vi "pixelfly_init.vi"(0 "trigger":bool=TRUE, 1 "V bin":i32(ring) items=["1", "2"], 2 "exp level":i32=1 min=0 max=255 step=1, 5 "Exposure mode":u16(ring)=1 items=["Asynch shutter", "Double shot", "Video mode", "Auto exposure"], 7 "exp time":i32=150 min=1 max=10000, 9 "gain":i32(ring) items=["Low (X1)", "High (X2)"], 11 "error in (no error)":errorcluster, 12 "H bin":i32(ring) items=["1", "2"]) -> (3 "X Bin":i32, 4 "boardid (indicator)":i32, 6 "Buffer number":i32, 8 "Buffer address":i32, 10 "Size":i32, 13 "initialized array":u8[][](array[numeric]), 14 "Y Bin":i32, 15 "error out":errorcluster)   [LabVIEW 2013]
doc: "Initializes the PixelFly camera and prepares it for 'pixelfly_acquire' to take images. Note that 'pixelfly_close' should be run when done imaging."
panel:
  in  "offset":i32
  # "Camera Controls"
  # "Camera Indicators"
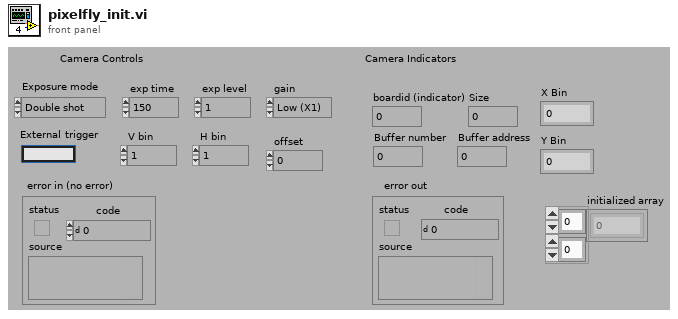
[diagram p1: front panel]
types:
  T1 = cluster{"ccdxsize":i32, "ccdy":i32, "pictx":i32, "picty":i32, "bitspixel":i32}
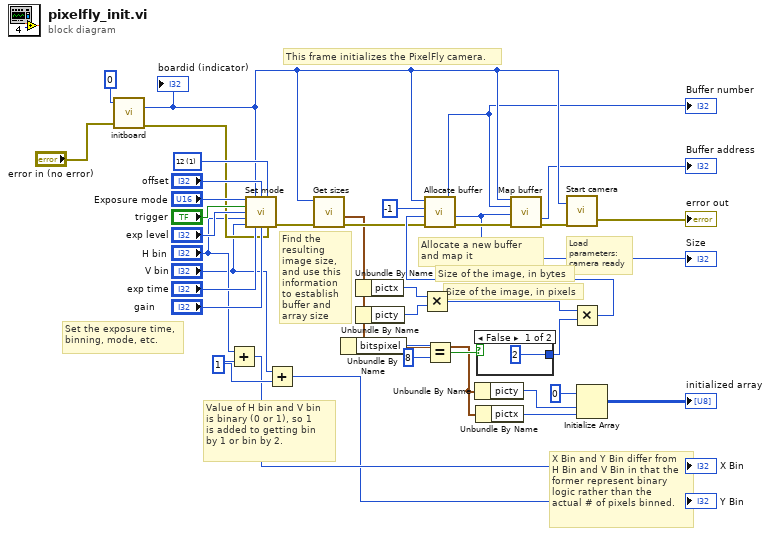
[diagram p0: block diagram]
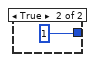
[diagram p2: hidden frame]
diagram:
  w9 = 1
  w19 = 1 items=["8", "12"] ("bits/pixel")
  # "Value of H bin and V bin\nis binary (0 or 1), so 1\nis added to getting bin\nby 1 or bin by 2."
  # "X Bin and Y Bin differ from\nH Bin and V Bin in that the\nformer represent binary\nlogic rather than the\nactual # of pixels binned."
  # "This frame initializes the PixelFly camera."
  # "Load parameters: camera ready"
  # "Allocate a new buffer and map it"
  # "Set the exposure time, binning, mode, etc."
  # "Find the resulting image size, and use this information to establish buffer and array size"
  # "Size of the image, in pixels"
  # "Size of the image, in bytes"
  n1 = call "initboard.vi"("boardid in"=0, "error in (no error)"="error in (no error)") -> ("boardid"=w12:i32, "error out"=w13:errorcluster)  [unwired: 2 in, 1 out]
  "boardid (indicator)" <- w12
  n2 = Add(x="H bin", y=w9) -> (x+y=→"X Bin":i32)
  n3 = call "Set mode.vi"("Exposure mode"="Exposure mode", "Handle in"=w12, "offset"="offset", "bits/pixel"=w19, "trigger"="trigger", "exp level"="exp level", "H bin"="H bin", "V bin"="V bin", "exp time"="exp time", "gain"="gain", "error in (no error)"=w13) -> ("error out"=w32:errorcluster)  [unwired: 4 in]
  n4 = Add(x="V bin", y=w9) -> (x+y=→"Y Bin":i32)
  n5 = call "Get sizes.vi"("Handle in"=w12, "error in (no error)"=w32) -> ("Picture parameters"=w18:T1, "error out"=w23:errorcluster)  [unwired: 1 in, 2 out]
  n6 = Unbundle By Name(w18) -> ("bitspixel"=w29:i32)
  n7 = Unbundle By Name(w18) -> ("pictx"=w31:i32)
  n8 = Unbundle By Name(w18) -> ("picty"=w30:i32)
  n9 = Multiply(x=w31, y=w30) -> (x*y=w26:i32)
  n10 = Equal?(x=w29, y=8) -> (x = y?=w27:bool)
  n11 = Unbundle By Name(w18) -> ("picty"=w16:i32)
  n12 = Unbundle By Name(w18) -> ("pictx"=w15:i32)
  n13 = case shown="False" w27 {
    tunnel: [2 1] -> w25
    frame False {
    }
    frame True {
    }
  }
  n14 = Multiply(x=w26, y=w25) -> (x*y=w24:i32)
  n15 = call "Allocate buffer.vi"("error in (no error)"=w23, "Size request"=w24, "Buffer request"=-1, "Handle in"=w12) -> ("error out"=w21:errorcluster, "Size"=w5:i32, "Buffer number"=w3:i32)  [unwired: 1 out]
  "Buffer number" <- w3
  "Size" <- w5
  n16 = call "Map buffer.vi"("Handle in"=w12, "Buffer in"=w3, "size"=w5, "error in (no error)"=w21) -> ("Buffer address"=→"Buffer address":i32, "error out"=w17:errorcluster)  [unwired: 8 in, 2 out]
  n17 = call "Start camera.vi"("Handle in"=w12, "error in (no error)"=w17) -> ("error out"=→"error out":errorcluster)  [unwired: 2 out]
  n18 = Initialize Array(u8 0 ("16 bit integers"), w16, w15) -> (→"initialized array":u8[][])
